vi "LabVIEW WEB.vi"() -> ()   [LabVIEW 2017]
uses:
  <vilib>/Instr/_visa.llb/VISA Configure Serial Port (Instr).vi
  <vilib>/httpClient/POSTBuffer.vi
  <vilib>/httpClient/LabVIEWHTTPClient.lvlib
panel:
  out "read buffer":string
  in  "VISA resource name":refnum<visa-resource-name>
  in  "stop":bool
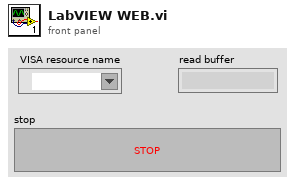
[diagram p1: front panel]
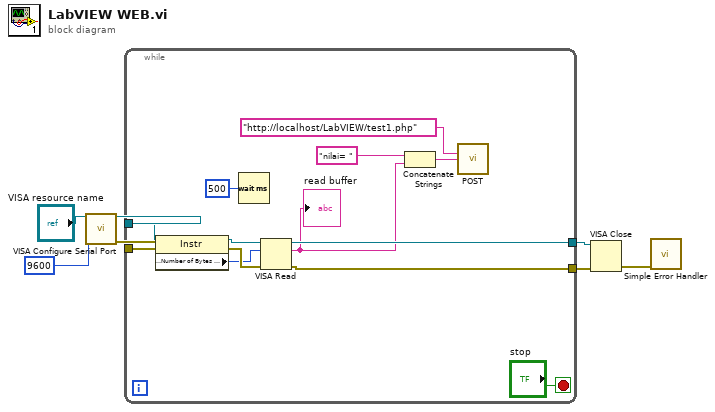
[diagram p0: block diagram]
diagram:
  n1 = call-poly "VISA Configure Serial Port"("VISA resource name"="VISA resource name", "baud rate (9600)"=u32 9600) -> ("VISA resource name out"=w6:refnum<visa-resource-name>, "error out"=w5:errorcluster)  [unwired: 12 in]
  n2 = while {
    tunnel: w6 -> [w19]
    tunnel: w5 -> [w18]
    tunnel: [w15] -> w3
    tunnel: [w14] -> w2
    stop <- "stop" stop-if-true
    n3 = property class="Instr"(reference=w19, error in=w18) -> (reference out=w17:refnum<visa-resource-name>, error out=w16:errorcluster, "Serial Settings:Number of Bytes at Serial Port"=w13:u32)
    n4 = Wait (ms)(milliseconds to wait=u32 500) -> ()  [unwired: 1 out]
    n5 = VISA Read(VISA resource name=w17, byte count=w13, error in (no error)=w16) -> (VISA resource name out=w15:refnum<visa-resource-name>, read buffer=w8:string, error out=w14:errorcluster)  [unwired: 1 out]
    "read buffer" <- w8
    n6 = Concatenate Strings("nilai= " ("string"), w8) -> (w9:string)
    n7 = call-poly <vilib>:"POST.vi"("url"="http://localhost/LabVIEW/test1.php", "buffer"=w9) -> ()  [unwired: 10 in, 4 out]
  }
  n8 = VISA Close(VISA resource name=w3, error in (no error)=w2) -> (error out=w1:errorcluster)
  n9 = call <vilib>:"Simple Error Handler.vi"("error in (no error)"=w1) -> ()  [unwired: 4 in, 5 out]
